vi "AboutScreen.vi"(11 "Version Info. In":string) -> ()   [LabVIEW 2020]
doc: "*-----------------------------------------------------\n* Author: SWatts\n*\n* VI Description: Displays About dialog\n* \n*\n* Error handling: All errors passed out\n*\n* Pre-condition: \n*\n* Post-condition: None\n*\n* Revision History:\n*\n* Rev Date Author Description \n* 01 30/04/2014 SWatts First issue\n*\n*-----------------------------------------------------"
uses:
  <vilib>/Platform/browser.llb/Open URL in Default Browser (string).vi
panel:
  in  "Website":bool
  in  "Close":bool
  out "Version Info.":string
  out "Version:":string
  # "Copyright 2020, SSDC Ltd"
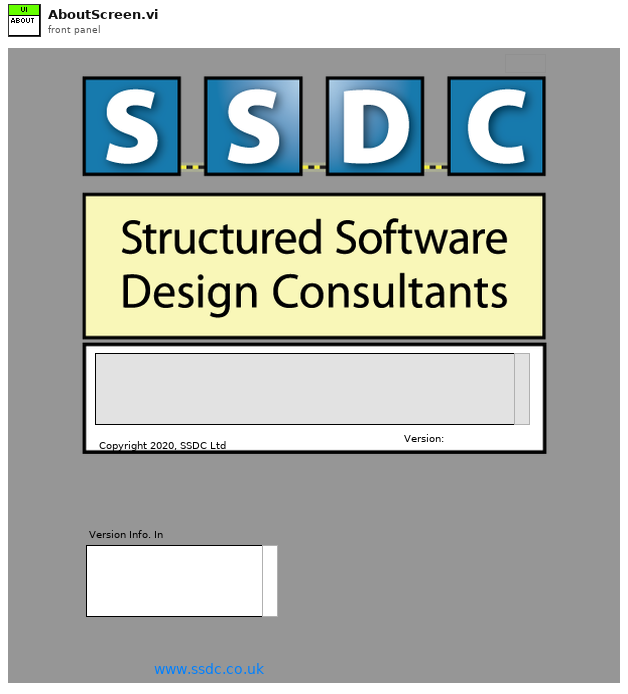
[diagram p1: front panel]
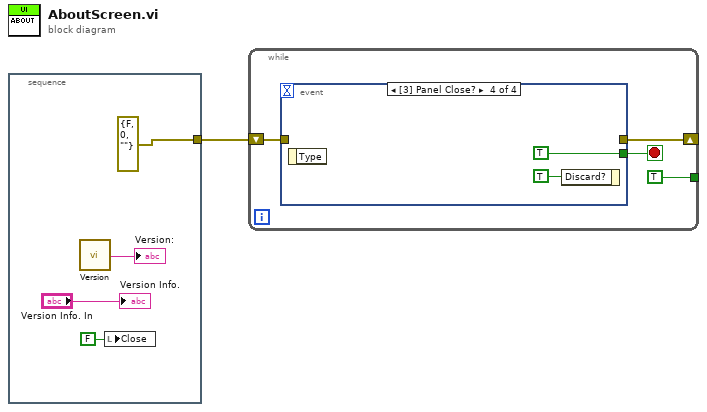
[diagram p0: block diagram]
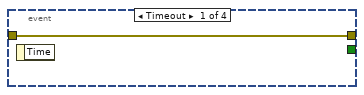
[diagram p2: hidden frame]
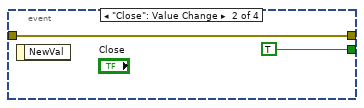
[diagram p3: hidden frame]
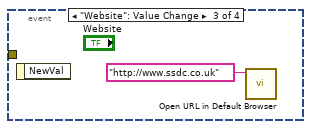
[diagram p4: hidden frame]
diagram:
  n1 = stacked-sequence {
    tunnel: [errorcluster {"status"=FALSE, "code"=0, "source"=""} ("error out")] -> w1
    frame #0 {
      n2 = call "Version.vi"() -> ("Version"=→"Version:":string)  [unwired: 5 in]
      n3 = local write "Close"(FALSE ("Close")) -> ()
      "Version Info." <- "Version Info. In"
    }
  }
  n4 = while {
    shift-right: [w9] -> _
    shift-left: w1 -> [w6]
    tunnel: [TRUE ("stop")] -> _
    stop <- w8 stop-if-true
    n5 = event shown="[3] Panel Close?" {
      selector: _ -> [_ _ _ _]
      dyn-events: _ -> [_ _ _ _]
      timeout: _ -> [_ _ _ _]
      tunnel: w6 -> [w10 w11 _ _]
      tunnel: [w10 w11 _ _] -> w9
      tunnel: [_ TRUE ("Close") _ TRUE ("Close")] -> w8
      event Timeout {
        n6 = event-data() -> ()  [unwired: 1 in, 1 out]
      }
      event "Close": Value Change {
        n7 = event-data() -> ()  [unwired: 1 in, 1 out]
      }
      event "Website": Value Change {
        n8 = event-data() -> ()  [unwired: 1 in, 1 out]
        n9 = call-poly <vilib>:"Open URL in Default Browser.vi"("URL"="http://www.ssdc.co.uk" ("Link")) -> ()  [unwired: 5 in, 2 out]
      }
      event Panel Close? {
        n10 = event-data() -> ()  [unwired: 1 in, 1 out]
        n11 = event-data("Discard?"=TRUE) -> ()  [unwired: 1 in, 1 out]
      }
    }
  }
